vi "ListenForConnection.vi"(8 "error in (no error)":errorcluster, 9 "timeout (2000 ms)":i32=2000, 11 "Listener":refnum<class "Connection.lvclass">) -> (0 "error out":errorcluster, 1 "New connection":bool, 2 "Connection":refnum<class "Connection.lvclass">, 3 "Listener out":refnum<class "Connection.lvclass">)   [LabVIEW 2013, in "MQTT_Connection.lvlib" / "Connection.lvclass"]
uses:
  Connection.lvclass
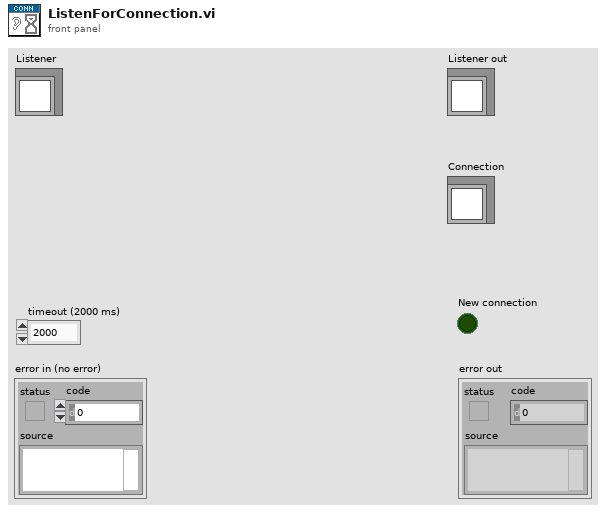
[diagram p1: front panel]
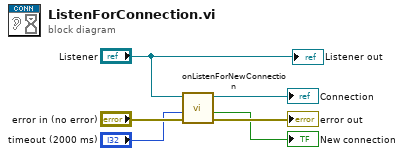
[diagram p0: block diagram]
diagram:
  n1 = call-dynamic "onListenForNewConnection.vi"("error in (no error)"="error in (no error)", "timeout (ms)"="timeout (2000 ms)", "Listener"="Listener") -> ("error out"=→"error out":errorcluster, "New connection"=→"New connection":bool, "New Connection"=→"Connection":refnum<class "Connection.lvclass">)  [unwired: 6 in]
  "Listener out" <- "Listener"
